vi "Get Theme Info.vi"(8 "Error In":errorcluster, 11 "ini Theme in":refnum<class "ini Theme.lvclass">) -> (0 "Error Out":errorcluster, 2 "Theme Info":T1, 3 "ini Theme out":refnum<class "ini Theme.lvclass">)   [LabVIEW 2021, in "Appearance Actor.lvlib" / "ini Theme.lvclass"]
doc: "Get theme informations such as <B>Name, Type (Light/Dark), Version, ...<B>."
uses:
  ini Theme.lvclass
  Generic Theme/API/Typedefs/Theme Info--cluster.ctl
  ini Theme.lvclass/ini Theme.ctl
  <vilib>/Utility/config.llb/Read Key (String).vi
  <vilib>/Utility/config.llb/NI_LVConfig.lvlib
  Generic Theme/Generic Theme.lvclass
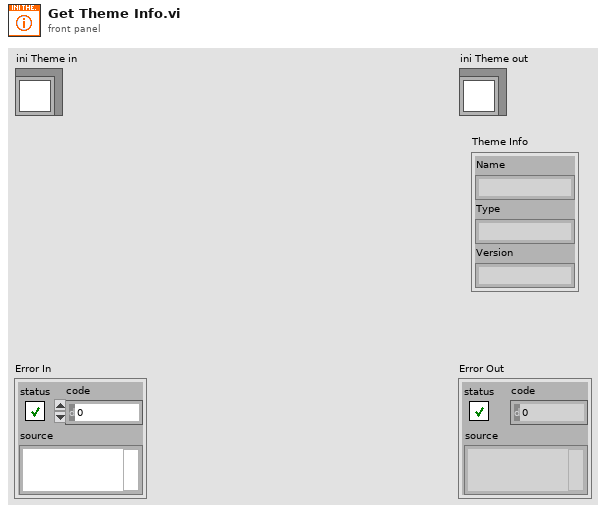
[diagram p1: front panel]
types:
  T1 = typedef "Appearance Actor.lvlib/Generic Theme.lvclass/Theme Info--cluster.ctl" = cluster{"Name":string, "Type":string, "Version":string}
  T2 = typedef "NI_LVConfig.lvlib/Config Data RefNum.ctl" = refnum<k1>
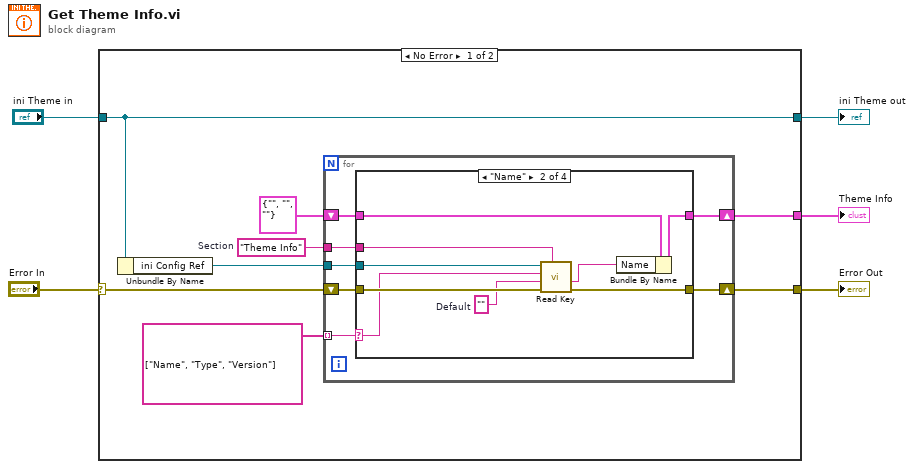
[diagram p0: block diagram]
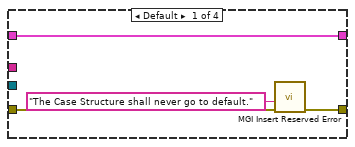
[diagram p2: hidden frame]
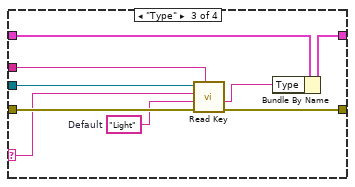
[diagram p3: hidden frame]
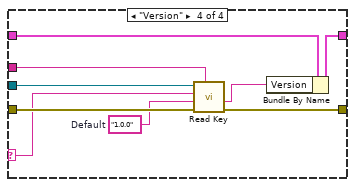
[diagram p4: hidden frame]
diagram:
  n1 = case shown="No Error" "Error In" {
    selector: "Error In" -> [w13 w53]
    tunnel: [w12 w53] -> w4
    tunnel: [w8 w52] -> w3
    tunnel: "ini Theme in" -> [w8 w52]
    tunnel: [w10 _] -> w1
    frame No Error {
      w9 = "Theme Info"  # Section
      n2 = Unbundle By Name(w8) -> ("ini Config Ref"=w7:T2)
      n3 = for {
        shift-right: [w19] -> w12
        shift-left: w13 -> [w20]
        shift-right: [w17] -> w10
        shift-left: T1 {"Name"="", "Type"="", "Version"=""} ("Theme Info") -> [w18]
        tunnel: w9 -> [w16]
        tunnel: w7 -> [w15]
        tunnel: string[] ["Name", "Type", "Version"] -> [w14] mode=indexing
        n4 = case shown="\"Name\"" w14 {
          selector: w14 -> [_ w28 w37 w46]
          tunnel: w20 -> [w23 w33 w42 w51]
          tunnel: [w22 w32 w41 w50] -> w19
          tunnel: w18 -> [w24 w31 w40 w49]
          tunnel: [w24 w27 w36 w45] -> w17
          tunnel: w16 -> [_ w30 w39 w48]
          tunnel: w15 -> [_ w29 w38 w47]
          frame Default {
            n5 = call <userlib>:"MGI Insert Reserved Error.vi"("Error In"=w23, "Error Description"="The Case Structure shall never go to default.") -> ("Error Out"=w22:errorcluster)  [unwired: 9 in]
          }
          frame "Name" {
            w25 = ""  # Default
            n6 = call-poly <vilib>:"Read Key.vi"("section"=w30, "error in (no error)"=w33, "default value"=w25, "key"=w28, "refnum"=w29) -> ("error out"=w32:errorcluster, "value"=w26:string)  [unwired: 3 in, 2 out]
            n7 = Bundle By Name(cluster=w31, "Name"=w26) -> (w27:T1)
          }
          frame "Type" {
            w34 = "Light"  # Default
            n8 = call-poly <vilib>:"Read Key.vi"("section"=w39, "error in (no error)"=w42, "default value"=w34, "key"=w37, "refnum"=w38) -> ("error out"=w41:errorcluster, "value"=w35:string)  [unwired: 3 in, 2 out]
            n9 = Bundle By Name(cluster=w40, "Type"=w35) -> (w36:T1)
          }
          frame "Version" {
            w43 = "1.0.0"  # Default
            n10 = call-poly <vilib>:"Read Key.vi"("section"=w48, "error in (no error)"=w51, "default value"=w43, "key"=w46, "refnum"=w47) -> ("error out"=w50:errorcluster, "value"=w44:string)  [unwired: 3 in, 2 out]
            n11 = Bundle By Name(cluster=w49, "Version"=w44) -> (w45:T1)
          }
        }
      }
    }
    frame Error {
    }
  }
  "Error Out" <- w4
  "ini Theme out" <- w3
  "Theme Info" <- w1
